vi "GraphXY.vi"() -> ()   [LabVIEW 2015]
uses:
  <vilib>/measure/NI_MABase.lvlib
panel:
  out "XY Graph":cluster{"Y":dbl[], "Y":dbl[]}(graph)
  in  "frequency 2":u8(knob)=10 scale=0.0..10.0
  in  "frequency":u8(knob)=10 scale=0.0..10.0
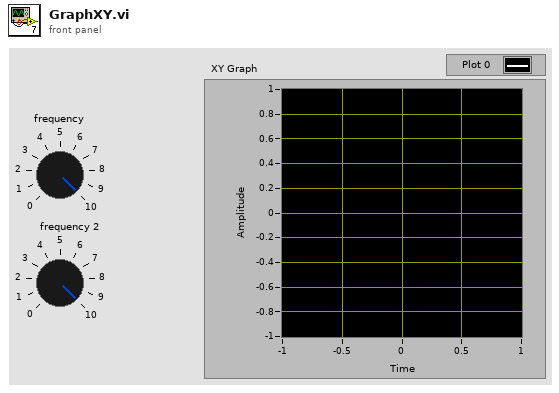
[diagram p1: front panel]
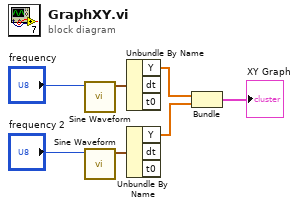
[diagram p0: block diagram]
diagram:
  n1 = call <vilib>:"Sine Waveform.vi"("frequency"="frequency") -> ("signal out"=w7:waveform(dbl))  [unwired: 9 in, 1 out]
  n2 = call <vilib>:"Sine Waveform.vi"("frequency"="frequency 2") -> ("signal out"=w4:waveform(dbl))  [unwired: 9 in, 1 out]
  n3 = Unbundle By Name(w7) -> ("Y"=w3:dbl[])  [unwired: 2 out]
  n4 = Unbundle By Name(w4) -> ("Y"=w2:dbl[])  [unwired: 2 out]
  n5 = Bundle("Y"=w3, "Y"=w2) -> (→"XY Graph":cluster{"Y":dbl[], "Y":dbl[]})  [unwired: 1 in]
